vi "Tracepoint_SendData.vi"(7 "Qbus in":refnum<class "Qbus.lvclass">, 8 "error in (no error)":errorcluster, 11 "data in":variant) -> (0 "error out":errorcluster)   [LabVIEW 2017, in "FileManager.lvlib"]
uses:
  <vilib>/addons/InsightCM/Devices/Shared/Common/FileManager/FileManager.lvlib
  <vilib>/addons/Qbus/Qbus.lvclass
  <vilib>/addons/TraceLogger/TraceLogger.lvlib
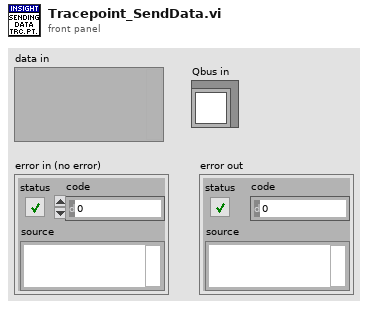
[diagram p1: front panel]
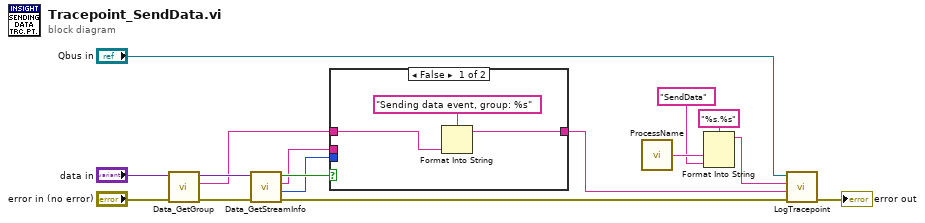
[diagram p0: block diagram]
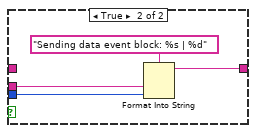
[diagram p2: hidden frame]
diagram:
  n1 = call <vilib>:"Data_GetGroup.vi"("error in"="error in (no error)", "data"="data in") -> ("error out"=w14:errorcluster, "data group"=w9:string, "data out"=w13:variant)  [unwired: 7 in]
  n2 = call <vilib>:"Data_GetStreamInfo.vi"("error in (no error)"=w14, "data"=w13) -> ("error out"=w7:errorcluster, "block"=w10:i32, "stream Id"=w11:string, "found"=w12:bool)  [unwired: 6 in]
  n3 = case shown="False" w12 {
    tunnel: w11 -> [_ w22]
    tunnel: w10 -> [_ w21]
    tunnel: [w18 w20] -> w5
    tunnel: w9 -> [w17 _]
    frame False {
      n4 = Format Into String(format string="Sending data event, group: %s", w17) -> (resulting string=w18:string)  [unwired: 2 in, 1 out]
    }
    frame True {
      n5 = Format Into String(format string="Sending data event block: %s | %d", w22, w21) -> (resulting string=w20:string)  [unwired: 2 in, 1 out]
    }
  }
  n6 = call <vilib>:"ProcessName.vi"() -> ("process name"=w4:string)  [unwired: 5 in]
  n7 = Format Into String(format string="%s.%s", w4, "SendData" ("tracepoint")) -> (resulting string=w1:string)  [unwired: 2 in, 1 out]
  n8 = call <vilib>:"LogTracepoint.vi"("error in (no error)"=w7, "log string"=w5, "tracepoint"=w1, "qbus in"="Qbus in") -> ("error out"=→"error out":errorcluster)  [unwired: 6 in, 1 out]
